vi "GenerateEvaporationString.vi"(10 "ODT Params":T1={"Waveform Parameters"=[[{"Initial Value"=1.2, "Final Value"=0.2, "Tau"=0.5, "Eta"=8.0, "Nickname"="Channel 0 A", "Enum"=enum."Evaporation Formula", "Conversion"=enum."Volts", "Constant"=0.0}, {"Initial Value"=5.0, "Final Value"=5.0, "Tau"=1.4, "Eta"=10.0, "Nickname"="Channel 0 B", "Enum"=enum."Evaporation Formula", "Conversion"=enum."Volts", "Constant"=0.0}, {"Initial Value"=0.0, "Final Value"=0.0, "Tau"=0.0, "Eta"=0.0, "Nickname"="Channel 0 C", "Enum"=enum."Power Law", "Conversion"=enum."Volts", "Constant"=0.0}, {"Initial Value"=0.0, "Final Value"=0.0, "Tau"=0.0, "Eta"=0.0, "Nickname"="Channel 0 D", "Enum"=enum."Power Law", "Conversion"=enum."Volts", "Constant"=0.0}], [{"Initial Value"=0.0, "Final Value"=0.0, "Tau"=0.0, "Eta"=0.0, "Nickname"="Channel 1 A", "Enum"=enum."Power Law", "Conversion"=enum."Volts", "Constant"=0.0}, {"Initial Value"=0.0, "Final Value"=0.0, "Tau"=0.0, "Eta"=0.0, "Nickname"="Channel 1 B", "Enum"=enum."Power Law", "Conversion"=enum."Volts", "Constant"=0.0}, {"Initial Value"=0.0, "Final Value"=0.0, "Tau"=0.0, "Eta"=0.0, "Nickname"="Channel 1 C", "Enum"=enum."Power Law", "Conversion"=enum."Volts", "Constant"=0.0}, {"Initial Value"=0.0, "Final Value"=0.0, "Tau"=0.0, "Eta"=0.0, "Nickname"="Channel 1 D", "Enum"=enum."Power Law", "Conversion"=enum."Volts", "Constant"=0.0}]], "Active Phases"=[TRUE, FALSE, FALSE, FALSE], "Active Channels"=[TRUE, FALSE], "Phase Times (s)"=[2.0, 1.0, 0.0, 0.0], "Active Device"="6221_ODT", "Trigger Channel"="/6221_ODT/PFI0", "Evaporation Phase"=0.0, "Evaporation Channel"=0.0} {"Evaporation Channel" min=0.0 max=1.0 step=1.0; "Evaporation Phase" min=0.0 max=4.0 step=1.0; "Phase Times (s)" format="%#_6p"}) -> (2 "ODT String":string)   [LabVIEW 2016]
uses:
  Neutral_DAQ/6221 arb waveforms/6221_panel.ctl
  Neutral_DAQ/6221 arb waveforms/6221_waveform_param.ctl
  6733_Red_MOT/Neutral_voltage_conversion_control.ctl
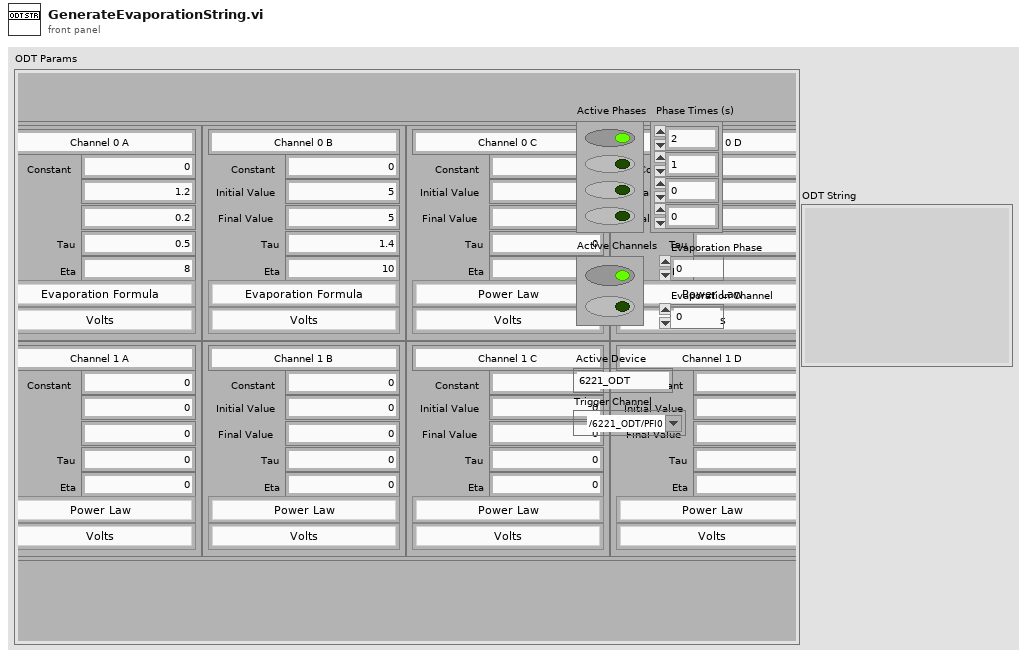
[diagram p1: front panel]
types:
  T1 = typedef "6221_panel.ctl" = cluster{"Waveform Parameters":T2[][], "Active Phases":bool[], "Active Channels":bool[], "Phase Times (s)":dbl[], "Active Device":string, "Trigger Channel":tag, "Evaporation Phase":dbl, "Evaporation Channel":dbl}
  T2 = typedef "6221_waveform_param.ctl" = cluster{"Initial Value":dbl, "Final Value":dbl, "Tau":dbl, "Eta":dbl, "Nickname":string, "Enum":enum16{"Power Law", "Evaporation Formula", "Evap - Calc Tau"}, "Conversion":T3, "Constant":dbl}
  T3 = typedef "Neutral_voltage_conversion_control.ctl" = enum16{"Volts", "B Field Grad (G/cm)", "Red Boson Cntr Freq (MHz)", "Red Boson Dither Amp (kHz)", "Red Boson Power (mW)", "Red 87 Trap Cntr Freq (MHz)", "Red 87 Trap Dither Amp (kHz)", "Red 87 Trap Power (mW)", "Red 87 Stir Cntr Freq (MHz)", "Red 87 Stir Dither Amp (kHz)", "Red 87 Stir Power (mW)", "ODT Sheet Trap Power (W)", "ODT Loading Trap Power (W)"}
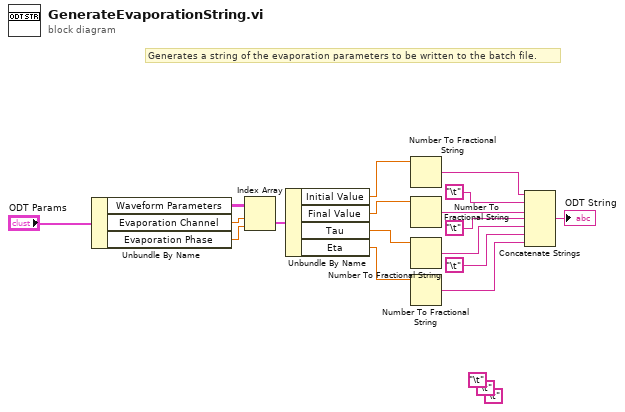
[diagram p0: block diagram]
diagram:
  (unwired) "\t"
  (unwired) "\t"
  (unwired) "\t"
  # "Generates a string of the evaporation parameters to be written to the batch file."
  n1 = Unbundle By Name("ODT Params") -> ("Waveform Parameters"=w16:T2[][], "Evaporation Channel"=w15:dbl, "Evaporation Phase"=w14:dbl)
  n2 = Index Array(array=w16, index (row)=w15, index (col)=w14) -> (element=w13:T2)
  n3 = Unbundle By Name(w13) -> ("Initial Value"=w12:dbl, "Final Value"=w9:dbl, "Tau"=w10:dbl, "Eta"=w11:dbl)
  n4 = Number To Fractional String(number=w12) -> (F-format string=w8:string)  [unwired: 3 in]
  n5 = Number To Fractional String(number=w9) -> (F-format string=w6:string)  [unwired: 3 in]
  n6 = Number To Fractional String(number=w10) -> (F-format string=w4:string)  [unwired: 3 in]
  n7 = Number To Fractional String(number=w11) -> (F-format string=w2:string)  [unwired: 3 in]
  n8 = Concatenate Strings(w8, "\t", w6, "\t", w4, "\t", w2) -> (→"ODT String":string)
